vi "Check Tolerance.vi"(1 "setpoint":dbl, 2 "Tolerance":dbl, 3 "Process variable":dbl) -> (0 "Boolean":bool)   [LabVIEW 2018]
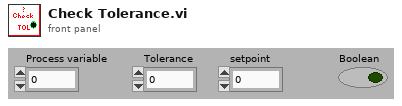
[diagram p1: front panel]
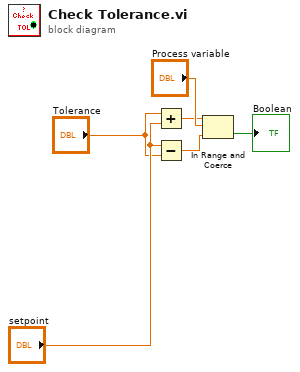
[diagram p0: block diagram]
diagram:
  n1 = Add(x="Tolerance", y="setpoint") -> (x+y=w3:dbl)
  n2 = Subtract(x="setpoint", y="Tolerance") -> (x-y=w2:dbl)
  n3 = In Range and Coerce(upper limit=w3, x="Process variable", lower limit=w2) -> (In Range?=→"Boolean":bool)  [unwired: 1 out]
